vi "editDialog.vi"(0 "reference":refnum<class "NoteNode.lvclass">, 1 "insidePackageNode":bool, 5 "error in (no error)":errorcluster) -> (14 "reference out":refnum<class "NoteNode.lvclass">, 15 "changeConnection":T1, 16 "cancel":bool, 19 "error out":errorcluster)   [LabVIEW 2012, in "NoteNode.lvclass"]
doc: "Edit Dialog"
uses:
  <resource>/Framework/Providers/Open_GDS/UML/NoteNode_class/NoteNode.lvclass
  <resource>/Framework/Providers/Open_GDS/UML/AbstractNode_class/private/NodeConnectionStatsType.ctl
  <vilib>/Utility/miscctls.llb/LVRectTypeDef.ctl
  <resource>/Framework/Providers/Open_GDS/UML/AbstractNode_class/AbstractNode.lvclass
  <resource>/Framework/Providers/Open_GDS/UML/MultiLineString_class/MultiLineString.lvclass
  <vilib>/event_ctls.llb/eventvkey.ctl
  <resource>/Framework/Providers/Open_GDS/UML/ContextHelp/ContextHelp_HelpTexts.ctl
  <vilib>/Utility/miscctls.llb/LVSelectionTypeDef.ctl
panel:
  in  "Underline":bool
  in  "Italic":bool
  in  "Bold":bool
  in  "Justify":u16(ring) items=["Left", "Center", "Right"]
  in  "Note color":u32(colorbox)
  in  "Help":bool
  in  "TextBox":string
  in  "connection":bool caption="Disconnect from Package"
  in  "OK Button":bool
  in  "Cancel Button":bool
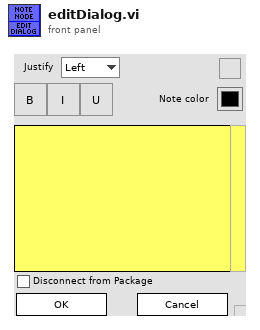
[diagram p1: front panel]
types:
  T1 = typedef "AbstractNode.lvclass/NodeConnectionStatsType.ctl" = enum16{"NA", "Connect", "DisConnect"}
  T2 = typedef "LVRectTypeDef.ctl" = cluster{"Left":i16, "Top":i16, "Right":i16, "Bottom":i16}
  T3 = cluster{"IgnoreStyleUpdate":bool, "Text":string, "Cancelled":bool, "InitSize":T2, "WidthChanged":bool}
  T4 = typedef "ContextHelp_HelpTexts.ctl" = enum16{"None(Hide)", "Default", "Help", "Welcome", "GettingStarted", "ClassDiagram_Help", "SequenceDiagram_Help", "UseCaseDiagram_Help", "BSelect", "BClass", "BInterface", "BPackage", "BNote", "BDependency", "BInheritance", "BInterfaceImplementation", "BAssociation", "BAggregation", "BCompAggregation", "BNoteConnector", "BObject", "BActionBar", "BCall", "BSystem", "BActor", "BUseCase", "BGeneralization", "BIncludes", "BExtends", "BUseCaseDiagramAssociation", "ClassRelationshipEdge editDialog_Bent Style", "ClassRelationshipEdge editDialog_RelationType", "ClassRelationshipEdge editDialog_Reverse association", "ClassRelationshipEdge editDialog_Start label", "ClassRelationshipEdge editDialog_Middle label", "ClassRelationshipEdge editDialog_End label", "UMLEditor reversedEngineering_Pathes", "ReversedEngineering StateReverseDialog_Help", "ReversedEngineering StateQueuedSettings_Help", "UMLEditor reversedEngineering_AddTopVIs", "UMLEditor reversedEngineering_AddClasses", "UMLEditor reversedEngineering_AddDirs", "UMLEditor reversedEngineering_Recursively", "UMLEditor reversedEngineering_Remove", "UMLEditor reversedEngineering_ClearList", "UMLEditor reversedEngineering_HideSubAss", "UMLEditor reversedEngineering_CreateTypes", "UMLEditor reversedEngineering_OnlyInheritance", "UMLEditor reversedEngineering_CreateApplication", "UMLEditor reversedEngineering_OK", "UMLEditor reversedEngineering_Cancel", "UMLEditor reversedEngineering_Help", "UMLEditor createWizardScriptFile_ScriptfilePath", "UMLEditor createWizardScriptFile_ClassPath", "UMLEditor createWizardScriptFile_Use", "UMLEditor createWizardScriptFile_PrivateDirName", "UMLEditor createWizardScriptFile_DirAppend", "UMLEditor createWizardScriptFile_Separator Character", "UMLEditor createWizardScriptFile_OK", "UMLEditor createWizardScriptFile_Cancel", "UMLEditor createWizardScriptFile_Help", "ClassNode editDialog_Class Name", "InterfaceNode editDialog_Class Name", "ClassNode editDialog_Attribute", "ClassNode editDialog_Methods", "InterfaceNode editDialog_Methods", "ClassNode editDialog_connection", "InterfaceNode editDialog_connection", "ClassNode editDialog_StereoType", "ClassNode editDialog_ShowAttrib", "ClassNode editDialog_ShowMethods", "ClassNode editDialog_ClassPath", "ClassNode editDialog_AddAttribute", "ClassNode editDialog_AddMethod", "InterfaceNode editDialog_AddMethod", "ClassNode AttributeGuide_AttributeName", "ClassNode AttributeGuide_Array?", "ClassNode AttributeGuide_Data Type", "ClassNode AttributeGuide_RefName", "ClassNode AttributeGuide_Preview", "ClassNode AttributeGuide_OK", "ClassNode AttributeGuide_Cancel", "ClassNode MethodGuide_Visibility", "ClassNode MethodGuide_Method Name", "ClassNode MethodGuide_Preview", "ClassNode MethodGuide_OK", "ClassNode MethodGuide_Cancel", "CallNode EditCallProperties_AllButtons", "ObjectNode EditObjectlProperties_AllButtons", "ActorNode EditActorProperties_AllButtons", "UseCaseRelationshipNode EditUseCaselProperties_AllButtons", "UseCaseNode EditUseCaselProperties_AllButtons", "SystemNode EditSystemProperties_AllButtons", "ReversedEngineering UpdateAttributes_AllButtons", "StateNode editDialog_AllButtons", "StateTransition editDialog_AllButtons", "ArrangeNodes Main_Picture", "ArrangeNodes Main_Zoom", "ArrangeNodes Main_Auto Zoom", "ArrangeNodes Main_shorten", "ArrangeNodes Main_Min Length", "ArrangeNodes Main_Max Length", "ArrangeNodes Main_increase", "ArrangeNodes Main_decrease", "ArrangeNodes Main_Shake", "ArrangeNodes Main", "BState", "BInitialState", "BFinalState", "BStateTransition", "StateDiagram_Help", "StateDiagram_PropertiesAllButtons", "ReversedEngineering StateReverseDialog_ClearStates", "ReversedEngineering StateReverseDialog_UseQueuedStateMachines", "ReversedEngineering StateReverseDialog_QueuedSettings", "ReversedEngineering StateReverseDialog_SearchForVIs", "ReversedEngineering StateReverseDialog_SearchCriteria", "OptionsDialog_ClassBasePath", "OptionsDialog_VIPath", "OptionsDialog_ApplicationPath", "OptionsDialog_WizDir", "OptionsDialog_IniFilePath", "OptionsDialog_DefineColors", "OptionsDialog_Help", "OptionsDialog_CreateTypes", "ClassRelationshipEdge editDialog_SplitWire"}
  T5 = typedef "LVSelectionTypeDef.ctl" = cluster{"Selection Start":u32, "Selection End":u32}
  T6 = typedef "NoteNode.lvclass/ObjectAttributes.ctl" = cluster{"Base class":T7, "DEFAULT_WIDTH":i32, "DEFAULT_HEIGHT":i32, "DEFAULT_COLOR":u32, "FOLD_X":i32, "FOLD_Y":i32, "color":u32, "text":refnum<class "MultiLineString.lvclass">, "pointNodes":refnum<class "AbstractNode.lvclass">[]}
  T7 = typedef "RectangularNode.lvclass/ObjectAttributes.ctl" = cluster{"Base class":T8, "bounds":T9}
  T8 = typedef "AbstractNode.lvclass/ObjectAttributes.ctl" = cluster{"parent":refnum<class "AbstractNode.lvclass">, "children":refnum<class "AbstractNode.lvclass">[], "Hidden":bool}
  T9 = typedef "Rectangle Rectangle2D.ctl" = cluster{"x":dbl, "y":dbl, "width":dbl, "height":dbl}
  T10 = typedef "MultiLineString.lvclass/JustificationType.ctl" = enum16{"LEFT", "CENTER", "RIGHT"}
  T11 = typedef "eventvkey.ctl" = enum16{"ASCII", "Enter", "Return", "Shift", "Ctrl", "Alt", "Cmd", "Opt", "Caps", "NumLock", "Clear", "Break", "Up", "Down", "Left", "Right", "Insert", "Delete", "Home", "End", "PageUp", "PageDown", "Escape", "Help", "Pause", "ScrollLock", "F1", "F2", "F3", "F4", "F5", "F6", "F7", "F8", "F9", "F10", "F11", "F12", "F13", "F14", "F15", "F16", "F17", "F18", "F19", "F20", "F21", "F22", "F23", "F24", "Play", "VolumeUp", "VolumeDown", "Mute", "Two Byte Char"}
  T12 = cluster{"Shift":bool, "Ctrl":bool, "Alt":bool, "Cmd":bool, "Opt":bool}
  T13 = typedef "ContextHelp_ShowType.ctl" = cluster{"Header":string, "Picture":picture, "Text":string}
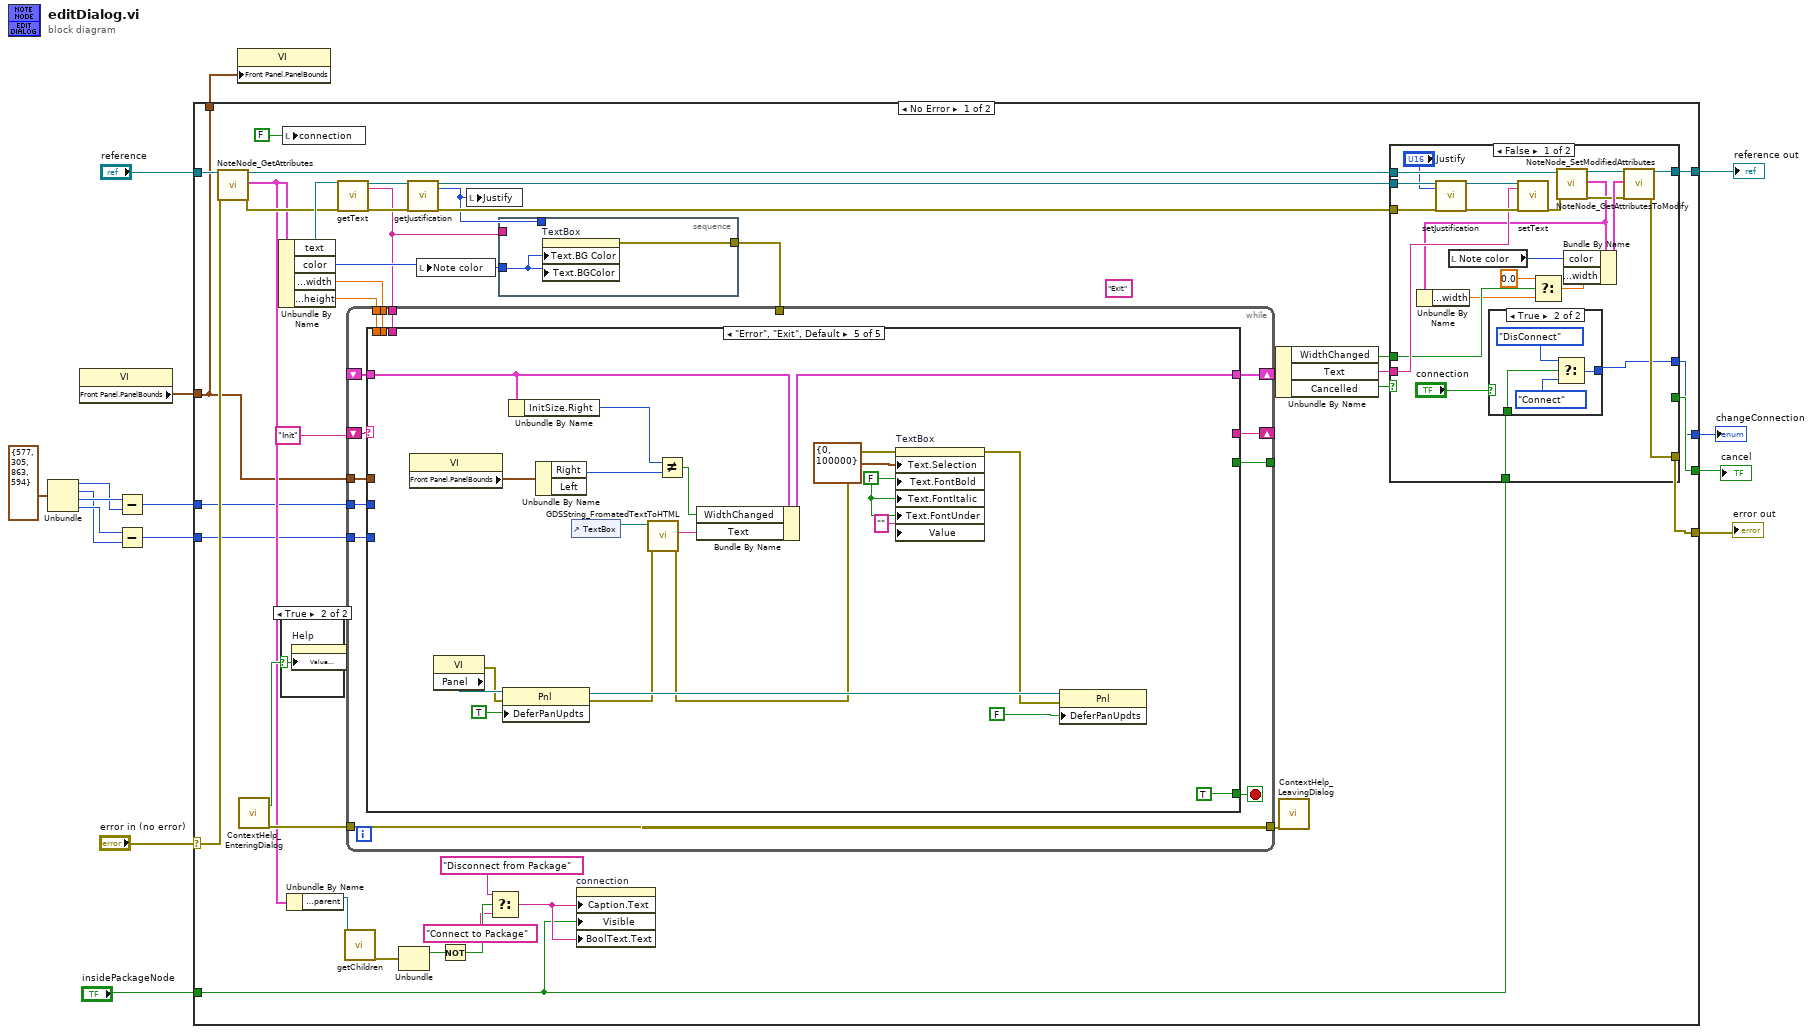
[diagram p0: block diagram]
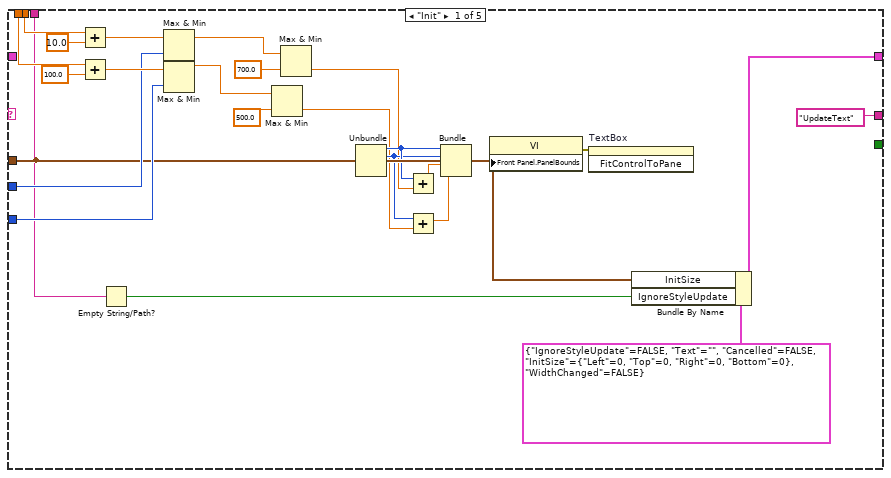
[diagram p3: hidden frame]
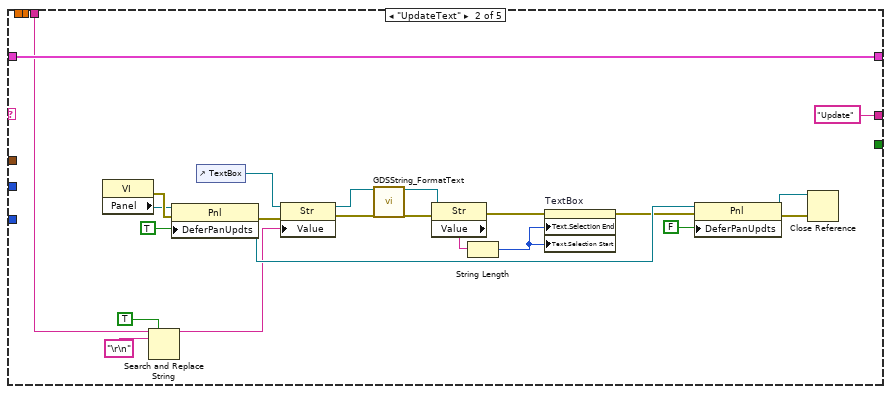
[diagram p4: hidden frame]
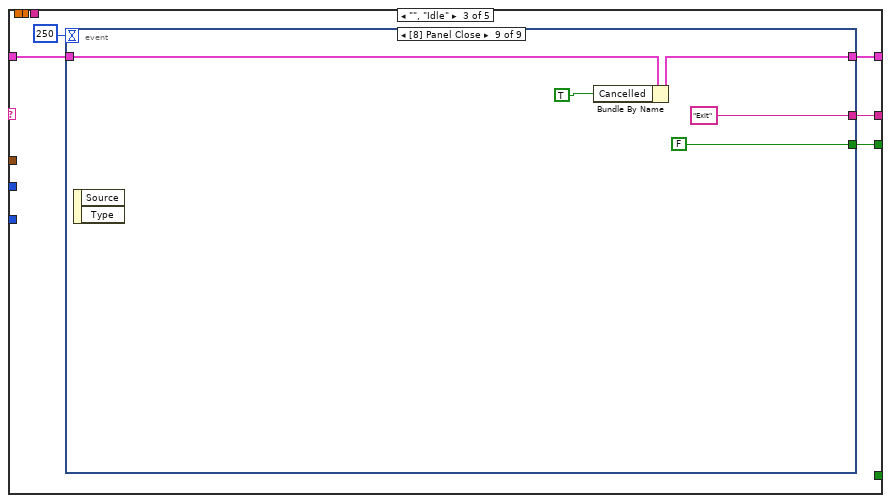
[diagram p5: hidden frame]
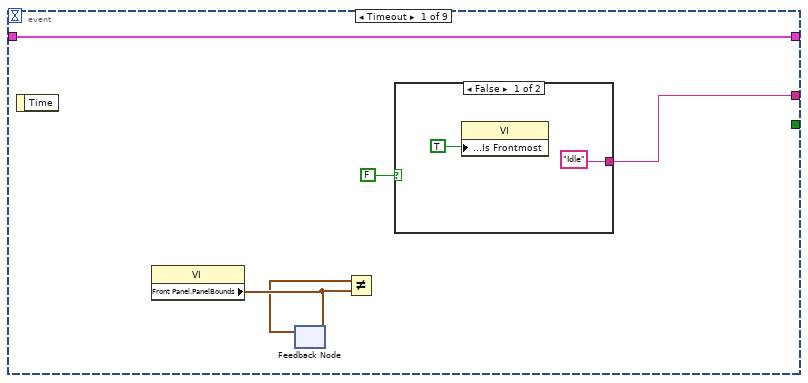
[diagram p6: hidden frame]
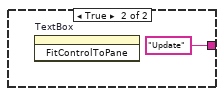
[diagram p7: hidden frame]
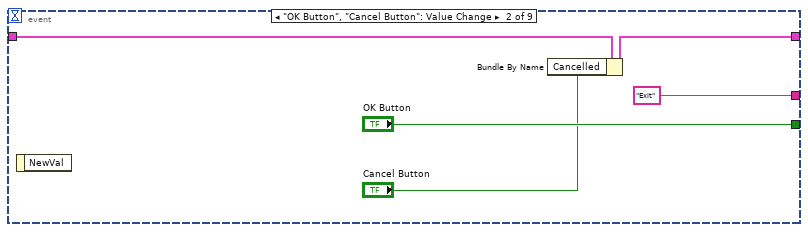
[diagram p8: hidden frame]
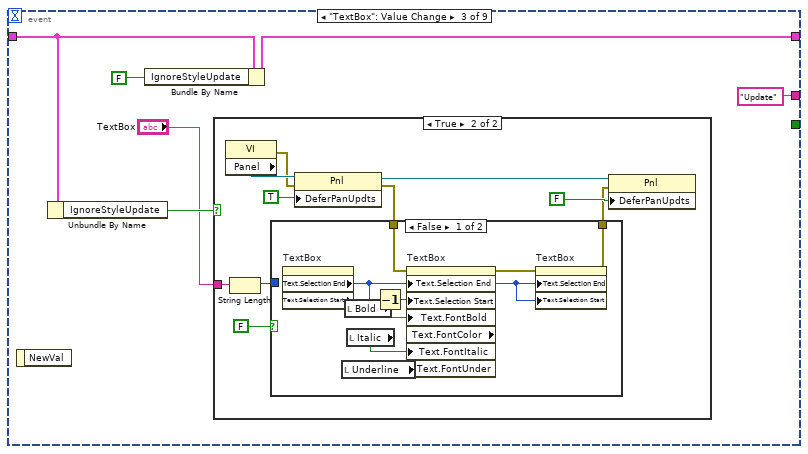
[diagram p9: hidden frame]
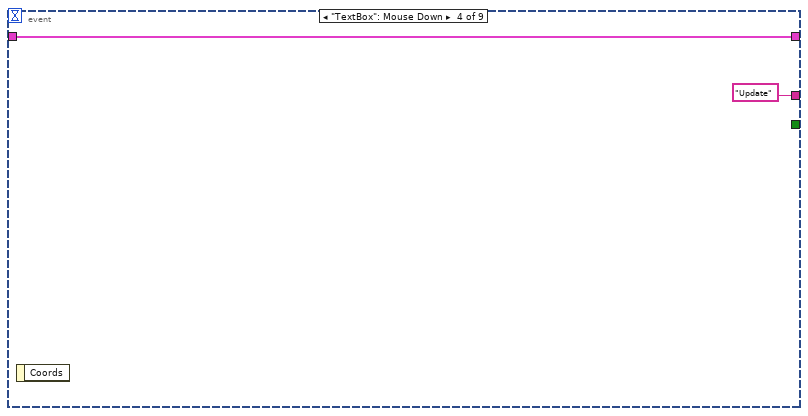
[diagram p12: hidden frame]
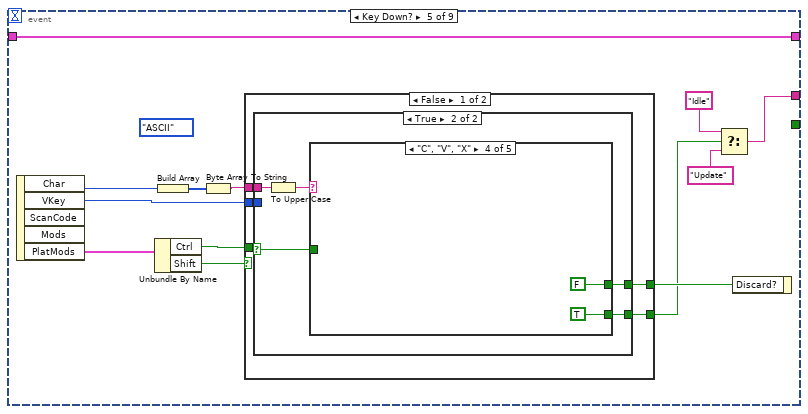
[diagram p13: hidden frame]
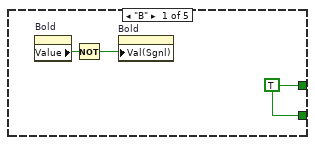
[diagram p16: hidden frame]
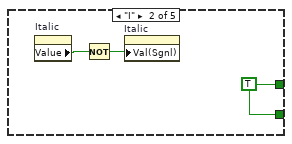
[diagram p17: hidden frame]
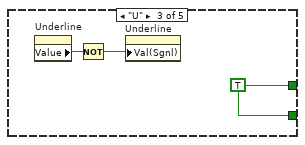
[diagram p18: hidden frame]
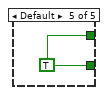
[diagram p19: hidden frame]
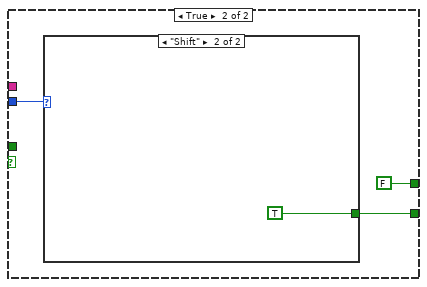
[diagram p20: hidden frame]
diagram:
  n1 = Unbundle(T2 {"Left"=577, "Top"=305, "Right"=863, "Bottom"=594} ("Front Panel Window:Panel Bounds")) -> ("Left"=w6:i16, "Top"=w4:i16, "Right"=w7:i16, "Bottom"=w5:i16)
  n2 = property class="VI"() -> ("Front Panel.PanelBounds"=w9:T2)  [unwired: 2 in, 2 out]
  n3 = Subtract(x=w7, y=w6) -> (x-y=w2:i16)
  n4 = Subtract(x=w5, y=w4) -> (x-y=w1:i16)
  n5 = case shown="No Error" "error in (no error)" {
    selector: "error in (no error)" -> [w51 w335]
    tunnel: "reference" -> [w52 w336]
    tunnel: [w56 w335] -> w14
    tunnel: [w55 w336] -> w13
    tunnel: [w48 TRUE ("Key Focus")] -> w12
    tunnel: [w39 _] -> w11
    tunnel: "insidePackageNode" -> [w31 _]
    tunnel: w9 -> [w20 w333]
    tunnel: [w20 w333] -> w3
    tunnel: w2 -> [w22 _]
    tunnel: w1 -> [w21 _]
    frame No Error {
      (unwired) "Exit"
      n6 = call <resource>:"NoteNode_GetAttributes.vi"("reference in"=w52, "error in (no error)"=w51) -> ("reference out"=w53:refnum<class "NoteNode.lvclass">, "Attributes"=w30:T6, "error out"=w49:errorcluster)  [unwired: 15 out]
      n7 = call <resource>:"ContextHelp_EnteringDialog.vi"() -> ("HelpStatus"=w45:bool, "error out"=w46:errorcluster)  [unwired: 3 in, 15 out]
      n8 = Unbundle By Name(w30) -> ("text"=w50:refnum<class "MultiLineString.lvclass">, "color"=w54:u32, "Base class.bounds.width"=w24:dbl, "Base class.bounds.height"=w23:dbl)
      n9 = case shown="True" w45 {
        selector: w45 -> [_ w57]
        frame False {
        }
        frame True {
          n10 = property on="Help" class="Bool (strict)"("Value (Signaling)"=w57) -> ()  [unwired: 2 in, 2 out]
        }
      }
      n11 = local write "connection"(FALSE ("connection")) -> ()
      n12 = Unbundle By Name(w30) -> ("Base class.Base class.parent"=w36:refnum<class "AbstractNode.lvclass">)
      n13 = call-dynamic "getText.vi"("reference"=w50, "error in (no error)"=w49) -> ("reference out"=w44:refnum<class "MultiLineString.lvclass">, "text"=w27:string, "error out"=w43:errorcluster)  [unwired: 15 in]
      n14 = call-dynamic "getChildren.vi"("reference"=w36) -> ("error out"=w34:errorcluster)  [unwired: 15 in, 3 out]
      n15 = Unbundle(w34) -> ("status"=w35:bool)  [unwired: 2 out]
      n16 = call <resource>:"getJustification.vi"("reference"=w44, "error in (no error)"=w43) -> ("reference out"=w41:refnum<class "MultiLineString.lvclass">, "justification"=w40:T10, "error out"=w42:errorcluster)  [unwired: 15 out]
      n17 = local write "Note color"(w54) -> ()
      n18 = Not(x=w35) -> (.not. x?=w37:bool)
      n19 = local write "Justify"(w40) -> ()
      n20 = Select(t="Disconnect from Package", s=w37, f="Connect to Package") -> (s? t:f=w38:string)
      n21 = stacked-sequence {
        tunnel: w54 -> [w332]
        tunnel: w27 -> [_]
        tunnel: w40 -> [_]
        tunnel: [w331] -> w19
        frame #0 {
          n22 = property on="TextBox" class="Str"("Text.BG Color"=w332, "Text.BGColor"=w332) -> (error out=w331:errorcluster)  [unwired: 2 in, 1 out]
        }
      }
      n23 = while {
        tunnel: [w70] -> _
        tunnel: [w68] -> w47
        tunnel: w46 -> [w68]
        shift-right: [w65] -> _
        shift-left: "Init" -> [w67]
        tunnel: w27 -> [w66]
        shift-right: [w64] -> w26
        shift-left: _ -> [w63]
        tunnel: w24 -> [w62]
        tunnel: w23 -> [w61]
        tunnel: w22 -> [w60]
        tunnel: w21 -> [w59]
        tunnel: w20 -> [w58]
        tunnel: w19 -> [_]
        stop <- w69 stop-if-true
        n24 = case shown="\"Error\", \"Exit\", Default" w67 {
          tunnel: [_ _ w124 _ _] -> w70
          tunnel: [_ _ _ _ TRUE ("Key Focus")] -> w69
          tunnel: w66 -> [w76 w101 _ _ _]
          tunnel: ["UpdateText" "Update" w122 _ _] -> w65
          tunnel: [w73 w110 w120 w233 w286] -> w64
          tunnel: w63 -> [_ w110 w121 w234 w285]
          tunnel: w62 -> [w95 _ _ _ _]
          tunnel: w61 -> [w94 _ _ _ _]
          tunnel: w60 -> [w89 _ _ _ _]
          tunnel: w59 -> [w88 _ _ _ _]
          tunnel: w58 -> [w87 _ _ _ _]
          frame "Init" {
            n25 = Add(x=w95, y=10.0) -> (x+y=w91:dbl)
            n26 = Add(x=w94, y=100.0) -> (x+y=w90:dbl)
            n27 = Empty String/Path?(string/path=w76) -> (empty?=w74:bool)
            n28 = Max & Min(x=w91, y=w89) -> (max(x,y)=w80:dbl)  [unwired: 1 out]
            n29 = Max & Min(x=w90, y=w88) -> (max(x,y)=w82:dbl)  [unwired: 1 out]
            n30 = Max & Min(x=w82, y=500.0) -> (min(x,y)=w81:dbl)  [unwired: 1 out]
            n31 = Max & Min(x=w80, y=700.0) -> (min(x,y)=w79:dbl)  [unwired: 1 out]
            n32 = Unbundle(w87) -> ("Left"=w86:i16, "Top"=w84:i16)  [unwired: 2 out]
            n33 = Add(x=w86, y=w79) -> (x+y=w85:dbl)
            n34 = Add(x=w84, y=w81) -> (x+y=w83:dbl)
            n35 = Bundle(cluster=w87, "Left"=w86, "Top"=w84, "Right"=w85, "Bottom"=w83) -> (w71:T2)
            n36 = property class="VI"("Front Panel.PanelBounds"=w71) -> (error out=w72:errorcluster)  [unwired: 2 in, 1 out]
            n37 = invoke on="TextBox" class="Str" method="FitControlToPane"(error in=w72) -> ()  [unwired: 2 in, 3 out]
            n38 = Bundle By Name(cluster=T3 {"IgnoreStyleUpdate"=FALSE, "Text"="", "Cancelled"=FALSE, "InitSize"={"Left"=0, "Top"=0, "Right"=0, "Bottom"=0}, "WidthChanged"=FALSE} ("State"), "InitSize"=w71, "IgnoreStyleUpdate"=w74) -> (w73:T3)
          }
          frame "UpdateText" {
            n39 = property class="VI"() -> (error out=w115:errorcluster, "Panel"=w113:refnum<vi>)  [unwired: 2 in, 1 out]
            n40 = Search and Replace String(replace all?=TRUE ("replace all? (F)"), input string=w101, search string="\r\n") -> (result string=w100:string)  [unwired: 5 in, 3 out]
            n41 = property class="Pnl"(reference=w113, error in=w115, "DeferPanUpdts"=TRUE ("Defer Panel Updates")) -> (reference out=w117:refnum<vi>, error out=w116:errorcluster)
            n42 = control-ref of="TextBox"() -> (w109:refnum<vi>)
            n43 = property on="Property Node" class="Str"(reference=w109, error in=w116, "Value"=w100) -> (reference out=w111:refnum<vi>, error out=w112:errorcluster)
            n44 = call <resource>:"GDSString_FormatText.vi"("TextIn"=w111, "error in"=w112) -> ("TextOut"=w108:refnum<vi>, "error out"=w107:errorcluster)  [unwired: 16 in]
            n45 = property on="Property Node" class="Str"(reference=w108, error in=w107) -> (error out=w106:errorcluster, "Value"=w105:string)  [unwired: 1 out]
            n46 = String Length(string=w105) -> (length=w102:i32)
            n47 = property on="TextBox" class="Str"(error in=w106, "Text.Selection End"=w102, "Text.Selection Start"=w102) -> (error out=w104:errorcluster)  [unwired: 1 in, 1 out]
            n48 = property class="Pnl"(reference=w117, error in=w104, "DeferPanUpdts"=FALSE ("Defer Panel Updates")) -> (reference out=w118:refnum<vi>, error out=w99:errorcluster)
            n49 = Close Reference(reference=w118, error in (no error)=w99) -> ()  [unwired: 1 out]
          }
          frame "", "Idle" {
            n50 = event shown="[8] Panel Close" {
              selector: _ -> [_ _ _ _ _ _ _ _ _]
              dyn-events: _ -> [_ _ _ _ _ _ _ _ _]
              timeout: 250 -> [_ _ _ _ _ _ _ _ _]
              tunnel: [_ "OK Button" _ _ _ _ _ _ FALSE ("OK Button")] -> w124
              tunnel: [w126 "Exit" "Update" "Update" w165 _ "Update" "Idle" "Exit"] -> w122
              tunnel: w121 -> [w129 w135 w140 w164 w177 w206 w212 w221 w230]
              tunnel: [w129 w134 w141 w164 w177 w206 w211 w221 w229] -> w120
              event Timeout {
                n51 = event-data() -> ()  [unwired: 2 out]
                n52 = property class="VI"() -> ("Front Panel.PanelBounds"=w128:T2)  [unwired: 2 in, 2 out]
                n53 = feedback-in #1(w128) -> ()
                n54 = feedback #1() -> (w127:T2)  [unwired: 1 in]
                n55 = Not Equal?(x=w127, y=w128) -> ()  [unwired: 1 out]
                n56 = case shown="False" FALSE {
                  tunnel: ["Idle" "Update"] -> w126
                  frame False {
                    n57 = property class="VI"("Front Panel Window:Is Frontmost"=TRUE) -> ()  [unwired: 2 in, 2 out]
                  }
                  frame True {
                    n58 = invoke on="TextBox" class="Str" method="FitControlToPane"() -> ()  [unwired: 3 in, 3 out]
                  }
                }
              }
              event "OK Button", "Cancel Button": Value Change {
                n59 = event-data() -> ()  [unwired: 2 out]
                n60 = Bundle By Name(cluster=w135, "Cancelled"="Cancel Button") -> (w134:T3)
              }
              event "TextBox": Value Change {
                n61 = event-data() -> ()  [unwired: 2 out]
                n62 = Unbundle By Name(w140) -> ("IgnoreStyleUpdate"=w143:bool)
                n63 = Bundle By Name(cluster=w140, "IgnoreStyleUpdate"=FALSE ("NewType")) -> (w141:T3)
                n64 = case shown="True" w143 {
                  tunnel: "TextBox" -> [_ w145]
                  frame False {
                  }
                  frame True {
                    n65 = property class="VI"() -> (error out=w151:errorcluster, "Panel"=w153:refnum<vi>)  [unwired: 2 in, 1 out]
                    n66 = String Length(string=w145) -> (length=w146:i32)
                    n67 = property class="Pnl"(reference=w153, error in=w151, "DeferPanUpdts"=TRUE ("Defer Panel Updates")) -> (reference out=w149:refnum<vi>, error out=w148:errorcluster)
                    n68 = case shown="False" FALSE {
                      tunnel: w146 -> [_ _]
                      tunnel: w148 -> [w160 w162]
                      tunnel: [w158 w162] -> w147
                      frame False {
                        n69 = property on="TextBox" class="Str" props=["Text", "Selection End", "Text", "Selection Start"]() -> ("Text.Selection End"=w154:u32)  [unwired: 2 in, 3 out]
                        n70 = local read "Underline"() -> (w155:bool)
                        n71 = local read "Bold"() -> (w157:bool)
                        n72 = local read "Italic"() -> (w156:bool)
                        n73 = Decrement(x=w154) -> (x-1=w161:u32)
                        n74 = property on="TextBox" class="Str" props=["Text", "Selection End", "Text", "Selection Start", "Text", "FontBold", "Text", "FontColor", "Text", "FontItalic", "Text", "FontUnder"](error in=w160, "Text.Selection End"=w154, "Text.Selection Start"=w161, "Text.FontBold"=w157, "Text.FontItalic"=w156, "Text.FontUnder"=w155) -> (error out=w159:errorcluster)  [unwired: 1 in, 2 out]
                        n75 = property on="TextBox" class="Str"(error in=w159, "Text.Selection End"=w154, "Text.Selection Start"=w154) -> (error out=w158:errorcluster)  [unwired: 1 in, 1 out]
                      }
                      frame True {
                      }
                    }
                    n76 = property class="Pnl"(reference=w149, error in=w147, "DeferPanUpdts"=FALSE ("Defer Panel Updates")) -> ()  [unwired: 2 out]
                  }
                }
              }
              event "TextBox": Mouse Down {
                n77 = event-data() -> ()  [unwired: 2 out]
              }
              event Key Down? {
                (unwired) eventvkey."ASCII" ("VKey")
                n78 = event-data() -> ("Char"=w172:i16, "VKey"=w171:T11, "PlatMods"=w170:T12)  [unwired: 3 out]
                n79 = Unbundle By Name(w170) -> ("Ctrl"=w174:bool, "Shift"=w173:bool)
                n80 = Build Array(w172) -> (w176:i16[])
                n81 = Byte Array To String(unsigned byte array=w176) -> (string=w175:string)
                n82 = case shown="False" w173 {
                  tunnel: w174 -> [w182 _]
                  tunnel: w175 -> [w181 _]
                  tunnel: [w180 FALSE ("Discard?")] -> w169
                  tunnel: [w179 w203] -> w168
                  tunnel: w171 -> [w178 w201]
                  frame False {
                    n83 = case shown="True" w182 {
                      selector: w182 -> [_ w186]
                      tunnel: w181 -> [_ w188]
                      tunnel: [_ w185] -> w180
                      tunnel: [_ w184] -> w179
                      tunnel: w178 -> [w183 _]
                      frame False {
                        n84 = case shown="\"ASCII\", Default" w183 {
                          frame "ASCII", Default {
                          }
                          frame "Home" {
                          }
                        }
                      }
                      frame True {
                        n85 = To Upper Case(1:w188) -> (0:w187:string)
                        n86 = case shown="\"C\", \"V\", \"X\"" w187 {
                          tunnel: w186 -> [_ _ _ _ _]
                          tunnel: [w189 w192 w195 FALSE ("Discard?") w200] -> w185
                          tunnel: [w189 w192 w195 TRUE ("Discard?") w200] -> w184
                          frame "B" {
                            w189 = TRUE ("Discard?")
                            n87 = property on="Bold" class="Bool (strict)"() -> ("Value"=w191:bool)  [unwired: 2 in, 2 out]
                            n88 = Not(x=w191) -> (.not. x?=w190:bool)
                            n89 = property on="Bold" class="Bool (strict)"("Val(Sgnl)"=w190) -> ()  [unwired: 2 in, 2 out]
                          }
                          frame "I" {
                            w192 = TRUE ("Discard?")
                            n90 = property on="Italic" class="Bool (strict)"() -> ("Value"=w194:bool)  [unwired: 2 in, 2 out]
                            n91 = Not(x=w194) -> (.not. x?=w193:bool)
                            n92 = property on="Italic" class="Bool (strict)"("Val(Sgnl)"=w193) -> ()  [unwired: 2 in, 2 out]
                          }
                          frame "U" {
                            w195 = TRUE ("Discard?")
                            n93 = property on="Underline" class="Bool (strict)"() -> ("Value"=w197:bool)  [unwired: 2 in, 2 out]
                            n94 = Not(x=w197) -> (.not. x?=w196:bool)
                            n95 = property on="Underline" class="Bool (strict)"("Val(Sgnl)"=w196) -> ()  [unwired: 2 in, 2 out]
                          }
                          frame "C", "V", "X" {
                          }
                          frame Default {
                            w200 = TRUE
                          }
                        }
                      }
                    }
                  }
                  frame True {
                    n96 = case shown="\"Shift\"" w201 {
                      tunnel: [_ TRUE] -> w203
                      frame Default {
                      }
                      frame "Shift" {
                      }
                    }
                  }
                }
                n97 = Select(t="Idle", s=w168, f="Update") -> (s? t:f=w165:string)
                n98 = event-data("Discard?"=w169) -> ()  [unwired: 1 in, 1 out]
              }
              event "Note color": Value Change {
                (unwired) "Idle"
                n99 = event-data() -> ()  [unwired: 2 out]
                n100 = property on="TextBox" class="Str"("Text.BG Color"="Note color", "Text.BGColor"="Note color") -> ()  [unwired: 2 in, 2 out]
              }
              event "Bold", "Italic", "Underline": Value Change {
                (unwired) TRUE ("Data Changed?")
                n101 = event-data() -> ()  [unwired: 2 out]
                n102 = property on="TextBox" class="Str"() -> ("Text.Selection End"=w217:u32, "Text.Selection Start"=w216:u32)  [unwired: 2 in, 2 out]
                n103 = local read "TextBox"() -> (w215:string)
                n104 = Equal?(x=w217, y=w216) -> (x = y?=w213:bool)
                n105 = String Length(string=w215) -> (length=w214:i32)
                n106 = case shown="False" w213 {
                  tunnel: "Bold" -> [w220 _]
                  tunnel: w214 -> [_ _]
                  tunnel: "Italic" -> [w219 _]
                  tunnel: "Underline" -> [w218 _]
                  frame False {
                    n107 = property on="TextBox" class="Str"("Text.FontUnder"=w218) -> ()  [unwired: 2 in, 2 out]
                    n108 = property on="TextBox" class="Str"("Text.FontBold"=w220) -> ()  [unwired: 2 in, 2 out]
                    n109 = property on="TextBox" class="Str"("Text.FontItalic"=w219) -> ()  [unwired: 2 in, 2 out]
                  }
                  frame True {
                  }
                }
                n110 = Bundle By Name(cluster=w212, "IgnoreStyleUpdate"=w213) -> (w211:T3)
              }
              event "Help": Value Change {
                n111 = event-data() -> ()  [unwired: 2 out]
                n112 = case shown="True" "Help" {
                  tunnel: [ContextHelp_HelpTexts."None(Hide)" ("HelpText") ContextHelp_HelpTexts."BNote" ("HelpText")] -> w224
                  frame False {
                  }
                  frame True {
                  }
                }
                n113 = call <resource>:"ContextHelp_HelpTexts.vi"("HelpText (enum or string)"=w224) -> ("HelpOut"=w225:T13)  [unwired: 18 out]
                n114 = call <resource>:"ContextHelp_SendMessageToPopUp.vi"("PopUpMessage"=w225) -> ()  [unwired: 2 in, 17 out]
              }
              event Panel Close {
                n115 = event-data() -> ()  [unwired: 3 out]
                n116 = Bundle By Name(cluster=w230, "Cancelled"=TRUE ("Key Focus")) -> (w229:T3)
              }
            }
          }
          frame "Update" {
            n117 = Unbundle By Name(w234) -> ("IgnoreStyleUpdate"=w235:bool)
            n118 = case shown="False" w235 {
              tunnel: [w243 _] -> w237
              tunnel: w234 -> [w239 w280]
              tunnel: [w239 w280] -> w233
              frame False {
                n119 = property on="TextBox" class="Str"() -> (error out=w244:errorcluster, "Text.Selection End"=w240:u32, "Text.Selection Start"=w241:u32)  [unwired: 2 in, 1 out]
                n120 = property class="VI"(error in=w244) -> (error out=w251:errorcluster, "Panel"=w253:refnum<vi>)  [unwired: 1 in, 1 out]
                n121 = Not Equal?(x=w240, y=w241) -> (x != y?=w242:bool)
                n122 = property class="Pnl"(reference=w253, error in=w251, "DeferPanUpdts"=TRUE ("Defer Panel Updates")) -> (reference out=w246:refnum<vi>, error out=w238:errorcluster)
                n123 = case shown="False" w242 {
                  tunnel: [w258 w277] -> w249
                  tunnel: [w259 w278] -> w248
                  tunnel: [w260 w279] -> w247
                  tunnel: w241 -> [w254 w273]
                  tunnel: w238 -> [w257 w275]
                  tunnel: [w255 w276] -> w245
                  tunnel: w240 -> [_ w272]
                  frame False {
                    n124 = case shown="Default" w254 {
                      selector: w254 -> [_ w265]
                      tunnel: [w261 w270] -> w260
                      tunnel: [w262 w269] -> w259
                      tunnel: [w263 w268] -> w258
                      tunnel: w257 -> [w264 w267]
                      tunnel: [w264 w266] -> w256
                      frame 0 {
                        n125 = local read "Underline"() -> (w261:bool)
                        n126 = local read "Bold"() -> (w263:bool)
                        n127 = local read "Italic"() -> (w262:bool)
                      }
                      frame Default {
                        n128 = Decrement(x=w265) -> (x-1=w271:u32)
                        n129 = property on="TextBox" class="Str" props=["Text", "Selection End", "Text", "Selection Start", "Text", "FontBold", "Text", "FontColor", "Text", "FontItalic", "Text", "FontUnder"](error in=w267, "Text.Selection End"=w265, "Text.Selection Start"=w271) -> (error out=w266:errorcluster, "Text.FontBold"=w268:bool, "Text.FontItalic"=w269:bool, "Text.FontUnder"=w270:bool)  [unwired: 1 in, 2 out]
                      }
                    }
                    n130 = property on="TextBox" class="Str"(error in=w256, "Text.Selection End"=w254, "Text.Selection Start"=w254) -> (error out=w255:errorcluster)  [unwired: 1 in, 1 out]
                  }
                  frame True {
                    n131 = property on="TextBox" class="Str"(error in=w275, "Text.Selection End"=w272, "Text.Selection Start"=w273) -> (error out=w274:errorcluster)  [unwired: 1 in, 1 out]
                    n132 = property on="TextBox" class="Str" props=["Text", "FontBold", "Text", "FontColor", "Text", "FontItalic", "Text", "FontUnder"](error in=w274) -> (error out=w276:errorcluster, "Text.FontBold"=w277:bool, "Text.FontItalic"=w278:bool, "Text.FontUnder"=w279:bool)  [unwired: 1 in, 2 out]
                  }
                }
                n133 = property class="Pnl"(reference=w246, error in=w245, "DeferPanUpdts"=FALSE ("Defer Panel Updates")) -> (error out=w243:errorcluster)  [unwired: 1 out]
                n134 = local write "Underline"(w247) -> ()
                n135 = local write "Bold"(w249) -> ()
                n136 = local write "Italic"(w248) -> ()
              }
              frame True {
              }
            }
            n137 = property on="TextBox" class="Str"(error in=w237, "Key Focus"=TRUE) -> ()  [unwired: 1 in, 2 out]
          }
          frame "Error", "Exit", Default {
            w293 = FALSE ("Text.Font:Bold")
            n138 = property class="VI"() -> ("Front Panel.PanelBounds"=w284:T2)  [unwired: 2 in, 2 out]
            n139 = property class="VI"() -> (error out=w297:errorcluster, "Panel"=w299:refnum<vi>)  [unwired: 2 in, 1 out]
            n140 = property class="Pnl"(reference=w299, error in=w297, "DeferPanUpdts"=TRUE ("Defer Panel Updates")) -> (reference out=w295:refnum<vi>, error out=w288:errorcluster)
            n141 = Unbundle By Name(w285) -> ("InitSize.Right"=w282:i16)
            n142 = Unbundle By Name(w284) -> ("Right"=w283:i16)  [unwired: 1 out]
            n143 = control-ref of="TextBox"() -> (w290:refnum<vi>)
            n144 = call <resource>:"GDSString_FromatedTextToHTML.vi"("error in (no error)"=w288, "FormattedStringIn"=w290) -> ("error out"=w287:errorcluster, "TextOut"=w289:string)  [unwired: 7 in, 1 out]
            n145 = Not Equal?(x=w282, y=w283) -> (x != y?=w281:bool)
            n146 = Bundle By Name(cluster=w285, "WidthChanged"=w281, "Text"=w289) -> (w286:T3)
            n147 = property on="TextBox" class="Str"(error in=w287, "Text.Selection"=T5 {"Selection Start"=0, "Selection End"=100000}, "Text.FontBold"=w293, "Text.FontItalic"=w293, "Text.FontUnder"=w293, "Value"="" ("TextBox")) -> (error out=w291:errorcluster)  [unwired: 1 in, 1 out]
            n148 = property class="Pnl"(reference=w295, error in=w291, "DeferPanUpdts"=FALSE ("Defer Panel Updates")) -> ()  [unwired: 2 out]
          }
        }
      }
      n149 = property on="connection" class="Bool (strict)"("Caption.Text"=w38, "Visible"=w31, "BoolText.Text"=w38) -> ()  [unwired: 2 in, 2 out]
      n150 = Unbundle By Name(w26) -> ("WidthChanged"=w17:bool, "Text"=w25:string, "Cancelled"=w18:bool)
      n151 = call <resource>:"ContextHelp_LeavingDialog.vi"("error in (no error)"=w47) -> ()  [unwired: 2 in, 17 out]
      n152 = case shown="False" w18 {
        tunnel: [w320 w329] -> w56
        tunnel: [w319 w330] -> w55
        tunnel: w53 -> [w318 w330]
        tunnel: w41 -> [w312 _]
        tunnel: w42 -> [w315 w329]
        tunnel: [_ TRUE ("Key Focus")] -> w48
        tunnel: [w309 _] -> w39
        tunnel: w31 -> [w308 _]
        tunnel: w25 -> [w307 _]
        tunnel: w17 -> [w304 _]
        frame False {
          n153 = call <resource>:"setJustification.vi"("reference"=w312, "justification"="Justify", "error in (no error)"=w315) -> ("reference out"=w313:refnum<class "MultiLineString.lvclass">, "error out"=w314:errorcluster)  [unwired: 15 out]
          n154 = local read "Note color"() -> (w306:u32)
          n155 = case shown="True" "connection" {
            tunnel: [enum16{"NA", "Connect", "DisConnect"}."NA" ("changeConnection") w326] -> w309
            tunnel: w308 -> [_ w327]
            frame False {
            }
            frame True {
              n156 = Select(t=enum16{"NA", "Connect", "DisConnect"}."DisConnect" ("changeConnection"), s=w327, f=enum16{"NA", "Connect", "DisConnect"}."Connect" ("changeConnection")) -> (s? t:f=w326:enum16{"NA", "Connect", "DisConnect"})
            }
          }
          n157 = call-dynamic "setText.vi"("reference"=w313, "text"=w307, "error in (no error)"=w314) -> ("error out"=w317:errorcluster)  [unwired: 15 in, 1 out]
          n158 = call <resource>:"NoteNode_GetAttributesToModify.vi"("reference in"=w318, "error in (no error)"=w317) -> ("reference out"=w322:refnum<class "NoteNode.lvclass">, "Attributes"=w305:T6, "error out"=w316:errorcluster)  [unwired: 1 in, 14 out]
          n159 = Unbundle By Name(w305) -> ("Base class.bounds.width"=w303:dbl)
          n160 = Select(t=0.0, s=w304, f=w303) -> (s? t:f=w302:dbl)
          n161 = Bundle By Name(cluster=w305, "color"=w306, "Base class.bounds.width"=w302) -> (w321:T6)
          n162 = call <resource>:"NoteNode_SetModifiedAttributes.vi"("reference in"=w322, "Attributes"=w321, "error in (no error)"=w316) -> ("reference out"=w319:refnum<class "NoteNode.lvclass">, "error out"=w320:errorcluster)  [unwired: 3 in, 12 out]
        }
        frame True {
        }
      }
    }
    frame Error {
    }
  }
  "reference out" <- w13
  "error out" <- w14
  "changeConnection" <- w11
  "cancel" <- w12
  n163 = property class="VI"("Front Panel.PanelBounds"=w3) -> ()  [unwired: 2 in, 2 out]
